vi "TickTockRefs.vi"() -> ()   [LabVIEW 2015]
panel:
  in  "Tock0Ref":refnum<k21>="Time0"
  in  "Tick0Ref":refnum<k21>="Time0"
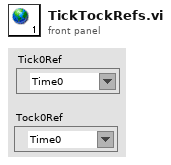
[diagram p1: front panel]
diagram:
